vi "TEST - Write Panel to INI.vi"(8 "error in (no error)":errorcluster) -> (0 "error out":errorcluster, 2 "Passed":bool)   [LabVIEW 2020]
uses:
  <userlib>/_OpenG.lib/file/file.llb/openg_file.lvlib
  <vilib>/Utility/config.llb/NI_LVConfig.lvlib
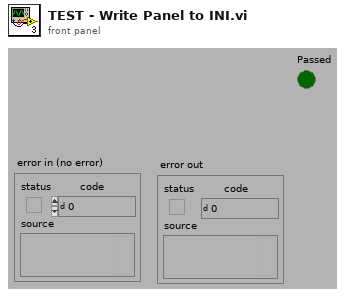
[diagram p1: front panel]
types:
  T1 = cluster{"label":string, "Variant":variant, "Variant":variant}
  T2 = typedef "NI_LVConfig.lvlib/Config Data RefNum.ctl" = refnum<k1>
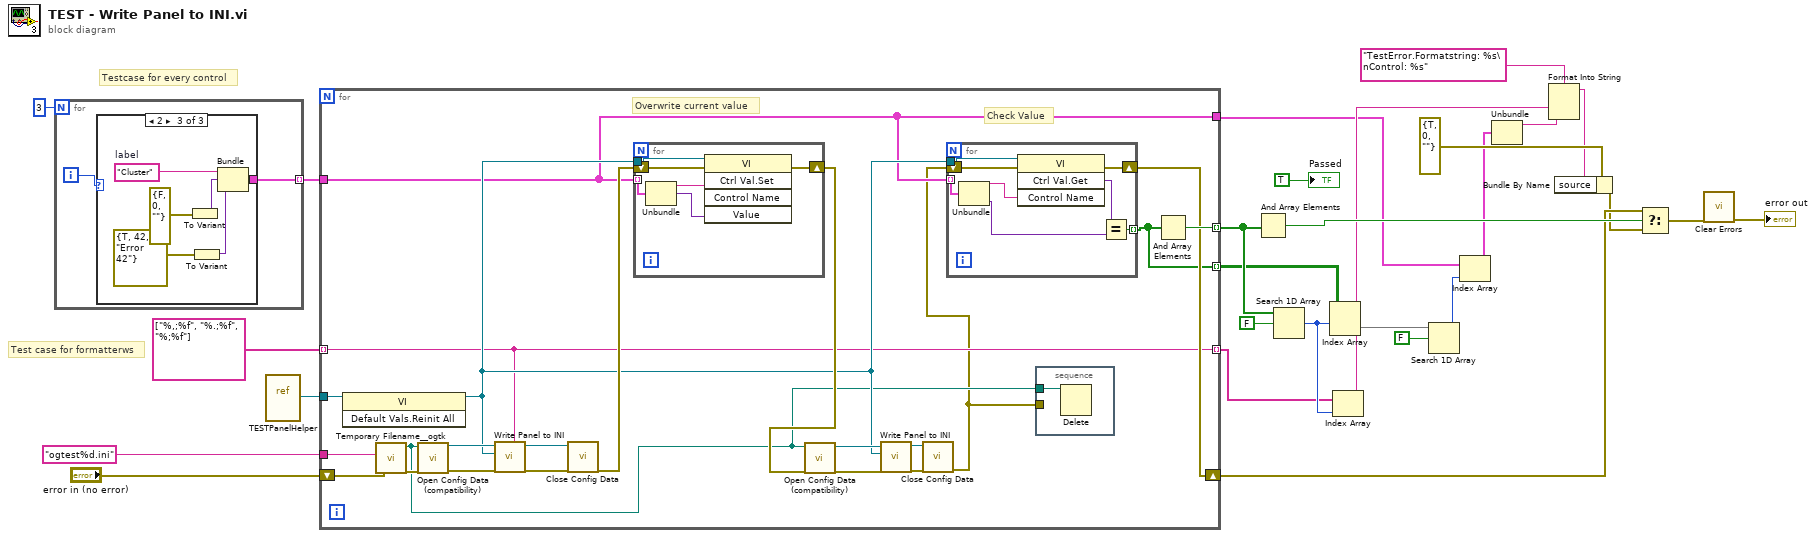
[diagram p0: block diagram]
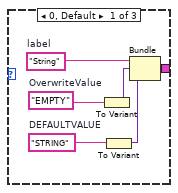
[diagram p2: hidden frame]
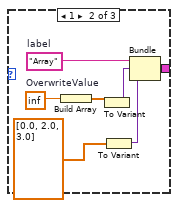
[diagram p3: hidden frame]
diagram:
  # "Test case for formatterws"
  # "Testcase for every control"
  n1 = for {
    N: 3 -> [_]
    tunnel: [w28] -> w22 mode=indexing
    i -> [w29]
    n2 = case shown="2" w29 {
      tunnel: [w30 w39 w45] -> w28
      frame 0, Default {
        w35 = "STRING"  # DEFAULTVALUE
        w34 = "EMPTY"  # OverwriteValue
        w33 = "String"  # label
        n3 = To Variant(anything=w34) -> (Variant=w32:variant)
        n4 = To Variant(anything=w35) -> (Variant=w31:variant)
        n5 = Bundle("label"=w33, "Variant"=w32, "Variant"=w31) -> (w30:T1)  [unwired: 1 in]
      }
      frame 1 {
        w36 = inf  # OverwriteValue
        w42 = "Array"  # label
        n6 = Build Array(w36) -> (w37:dbl[])
        n7 = To Variant(anything=w37) -> (Variant=w41:variant)
        n8 = To Variant(anything=dbl[] [0.0, 2.0, 3.0] ("Array")) -> (Variant=w40:variant)
        n9 = Bundle("label"=w42, "Variant"=w41, "Variant"=w40) -> (w39:T1)  [unwired: 1 in]
      }
      frame 2 {
        w48 = "Cluster"  # label
        n10 = To Variant(anything=errorcluster {"status"=FALSE, "code"=0, "source"=""} ("Cluster")) -> (Variant=w47:variant)
        n11 = To Variant(anything=errorcluster {"status"=TRUE, "code"=42, "source"="Error 42"} ("Cluster")) -> (Variant=w46:variant)
        n12 = Bundle("label"=w48, "Variant"=w47, "Variant"=w46) -> (w45:T1)  [unwired: 1 in]
      }
    }
  }
  n13 = vi-ref "TESTPanelHelper.vi"() -> (w25:refnum<vi>)
  n14 = for {
    tunnel: "ogtest%d.ini" ("pattern (lvtemp%d.tmp)") -> [w70]
    tunnel: w25 -> [w67]
    shift-right: [w54] -> w13
    shift-left: "error in (no error)" -> [w69]
    tunnel: string[] ["%,;%f", "%.;%f", "%;%f"] -> [w52] mode=indexing
    tunnel: w22 -> [w51]
    tunnel: [w55] -> w21 mode=indexing
    tunnel: [w53] -> w19 mode=indexing
    tunnel: [w52] -> w15 mode=indexing
    tunnel: [w51] -> w9
    # "Check Value"
    # "Overwrite current value"
    n15 = invoke class="VI" method="Default Vals.Reinit All"(reference=w67) -> (reference out=w56:refnum<vi>)  [unwired: 2 in, 2 out]
    n16 = call <userlib>:"Temporary Filename__ogtk.vi"("error in (no error)"=w69, "pattern (lvtemp%d.tmp)"=w70) -> ("error out"=w68:errorcluster, "file in tmp dir"=w50:path)  [unwired: 4 in]
    n17 = call <vilib>:"Open Config Data (compatibility).vi"("error in (no error)"=w68, "configuration file path"=w50) -> ("error out"=w66:errorcluster, "refnum"=w65:T2)  [unwired: 7 in, 1 out]
    n18 = call "Write Panel to INI.vi"("float number format (optional)"=w52, "error in (no error)"=w66, "VI ref"=w56, "refnum"=w65) -> ("error out"=w63:errorcluster, "refnum out"=w64:T2)  [unwired: 6 in]
    n19 = call <vilib>:"Close Config Data.vi"("error in (no error)"=w63, "refnum"=w64) -> ("error out"=w62:errorcluster)  [unwired: 8 in, 1 out]
    n20 = for {
      tunnel: w51 -> [w84] mode=indexing
      tunnel: w56 -> [w85]
      shift-right: [w80] -> w61
      shift-left: w62 -> [w81]
      n21 = Unbundle(w84) -> ("label"=w83:string, "Variant"=w82:variant)  [unwired: 1 out]
      n22 = invoke class="VI" method="Ctrl Val.Set"(reference=w85, error in=w81, "Control Name"=w83, "Value"=w82) -> (error out=w80:errorcluster)  [unwired: 1 in, 4 out]
    }
    n23 = call <vilib>:"Open Config Data (compatibility).vi"("error in (no error)"=w61, "configuration file path"=w50) -> ("error out"=w59:errorcluster, "refnum"=w60:T2)  [unwired: 7 in, 1 out]
    n24 = call "Write Panel to INI.vi"("error in (no error)"=w59, "VI ref"=w56, "refnum"=w60) -> ("error out"=w57:errorcluster, "refnum out"=w58:T2)  [unwired: 7 in]
    n25 = call <vilib>:"Close Config Data.vi"("error in (no error)"=w57, "refnum"=w58) -> ("error out"=w49:errorcluster)  [unwired: 8 in, 1 out]
    n26 = for {
      tunnel: w51 -> [w78] mode=indexing
      tunnel: w56 -> [w79]
      shift-right: [w76] -> w54
      shift-left: w49 -> [w77]
      tunnel: [w72] -> w53 mode=indexing
      n27 = Unbundle(w78) -> ("label"=w75:string, "Variant"=w73:variant)  [unwired: 1 out]
      n28 = invoke class="VI" method="Ctrl Val.Get"(reference=w79, error in=w77, "Control Name"=w75) -> (error out=w76:errorcluster, "Get Control Value Variant"=w74:variant)  [unwired: 1 in, 2 out]
      n29 = Equal?(x=w74, y=w73) -> (x = y?=w72:bool)
    }
    n30 = stacked-sequence {
      tunnel: w50 -> [w71]
      tunnel: w49 -> [_]
      frame #0 {
        n31 = Delete(path (use dialog)=w71) -> ()  [unwired: 4 in, 3 out]
      }
    }
    n32 = And Array Elements(Boolean array=w53) -> (logical AND=w55:bool)
  }
  n33 = And Array Elements(Boolean array=w21) -> (logical AND=w14:bool)
  n34 = Search 1D Array(1D array=w21, element=FALSE) -> (index of element=w16:i32)  [unwired: 1 in]
  n35 = Index Array(array=w19, index (row)=w16) -> (element=w17:bool[])  [unwired: 1 in]
  n36 = Index Array(array=w15, index=w16) -> (element=w10:string)
  n37 = Search 1D Array(1D array=w17, element=FALSE) -> (index of element=w8:i32)  [unwired: 1 in]
  n38 = Index Array(array=w9, index=w8) -> (element=w7:T1)
  n39 = Unbundle(w7) -> ("label"=w6:string)  [unwired: 2 out]
  n40 = Format Into String(format string="TestError.Formatstring: %s\nControl: %s", w10, w6) -> (resulting string=w4:string)  [unwired: 2 in, 1 out]
  n41 = Bundle By Name(cluster=errorcluster {"status"=TRUE, "code"=0, "source"=""} ("t"), "source"=w4) -> (w5:errorcluster)
  n42 = Select(t=w13, s=w14, f=w5) -> (s? t:f=w2:errorcluster)
  n43 = call <vilib>:"Clear Errors.vi"("error in (no error)"=w2) -> ("error out"=→"error out":errorcluster)  [unwired: 5 in, 1 out]
  "Passed" <- TRUE ("Passed")
